vi "RichToFlatgoogle_protobuf_Timestamp.vi"(5 "OutputClusterType":T1, 11 "InputCluster":T2) -> (3 "OutputCluster":T1)   [LabVIEW 2025, in "bus_monitor_server.lvlib"]
uses:
  bus_monitor_server.lvlib
  google_protobuf_Timestamp.ctl
  google_protobuf_Timestamp_Flat.ctl
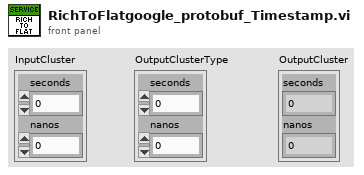
[diagram p1: front panel]
types:
  T1 = typedef "bus_monitor_server.lvlib/google_protobuf_Timestamp_Flat.ctl" = cluster{"seconds":i64, "nanos":i32}
  T2 = typedef "bus_monitor_server.lvlib/google_protobuf_Timestamp.ctl" = cluster{"seconds":i64, "nanos":i32}
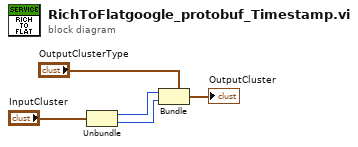
[diagram p0: block diagram]
diagram:
  n1 = Unbundle "Unbundle"("InputCluster") -> ("seconds"=w2:i64, "nanos"=w1:i32)
  n2 = Bundle "Bundle"(cluster="OutputClusterType", "seconds"=w2, "nanos"=w1) -> (→"OutputCluster":T1)
